vi "QVA_DestroyQueue.vi"(0 "QueueIn":refnum<queue>, 3 "ForceDestroy":bool=TRUE, 5 "ErrorIn":errorcluster) -> (15 "QueueName":string, 17 "ElementInQueue":variant[](array[variant]), 19 "ErrorOut":errorcluster)   [LabVIEW 2016]
doc: "Zerstört eine QVA\n\nsige / 3.12.13"
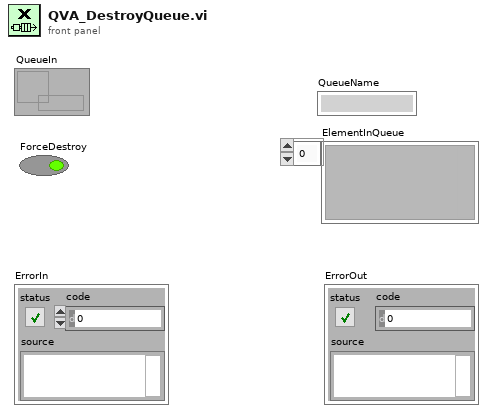
[diagram p1: front panel]
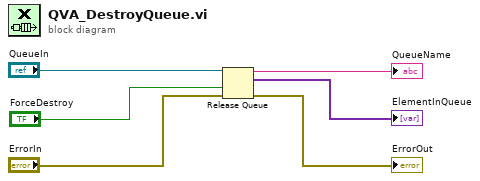
[diagram p0: block diagram]
diagram:
  n1 = Release Queue(queue="QueueIn", force destroy? (F)="ForceDestroy", error in (no error)="ErrorIn") -> (queue name=→"QueueName":string, remaining elements=→"ElementInQueue":variant[], error out=→"ErrorOut":errorcluster)
